vi "StripNLevelsAndBuildPath.vi"(5 "Create Folders":bool, 6 "Build Path":string, 7 "Strip Levels":i32=1, 8 "error in(no error)":errorcluster, 10 "Is File":bool, 11 "Path In":path) -> (0 "error out":errorcluster, 3 "Path Out":path)   [LabVIEW 2011]
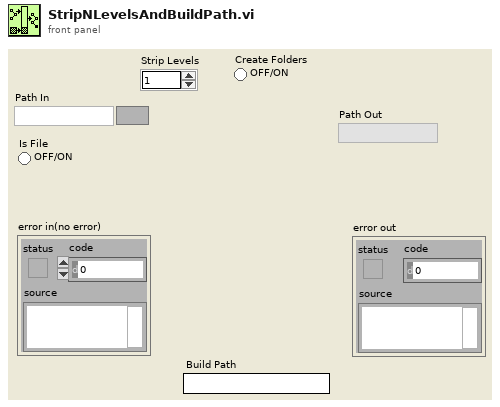
[diagram p1: front panel]
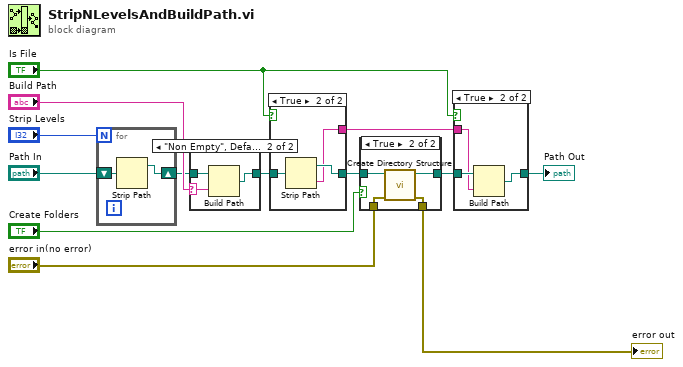
[diagram p0: block diagram]
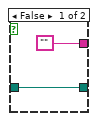
[diagram p3: hidden frame]
diagram:
  n1 = for {
    N: "Strip Levels" -> [_]
    shift-right: [w15] -> w7
    shift-left: "Path In" -> [w14]
    n2 = Strip Path(path=w14) -> (stripped path=w15:path)  [unwired: 1 out]
  }
  n3 = case shown="\"Non Empty\", Default" "Build Path" {
    selector: "Build Path" -> [_ w17]
    tunnel: w7 -> [w16 w19]
    tunnel: [w16 w18] -> w6
    frame "" {
    }
    frame "Non Empty", Default {
      n4 = Build Path(base path=w19, name or relative path=w17) -> (appended path=w18:path)
    }
  }
  n5 = case shown="True" "Is File" {
    tunnel: w6 -> [w21 w24]
    tunnel: [w21 w23] -> w5
    tunnel: ["" w22] -> w2
    frame False {
    }
    frame True {
      n6 = Strip Path(path=w24) -> (stripped path=w23:path, name=w22:string)
    }
  }
  n7 = case shown="True" "Create Folders" {
    tunnel: w5 -> [w25 w30]
    tunnel: [w25 w29] -> w3
    tunnel: "error in(no error)" -> [w26 w28]
    tunnel: [w26 w27] -> w9
    frame False {
    }
    frame True {
      n8 = call "Create Directory Structure.vi"("error in(no error)"=w28, "Dir Path In"=w30) -> ("error out"=w27:errorcluster, "Dir Path Out"=w29:path)  [unwired: 8 out]
    }
  }
  "error out" <- w9
  n9 = case shown="True" "Is File" {
    tunnel: w3 -> [w31 w34]
    tunnel: w2 -> [_ w33]
    tunnel: [w31 w32] -> w1
    frame False {
    }
    frame True {
      n10 = Build Path(base path=w34, name or relative path=w33) -> (appended path=w32:path)
    }
  }
  "Path Out" <- w1
